vi "FT10_Log Tester Queue Data.vi"(10 "Queue in":refnum<queue>, 11 "Cluster in":T1) -> (3 "Cluster out":T1)   [LabVIEW 2015]
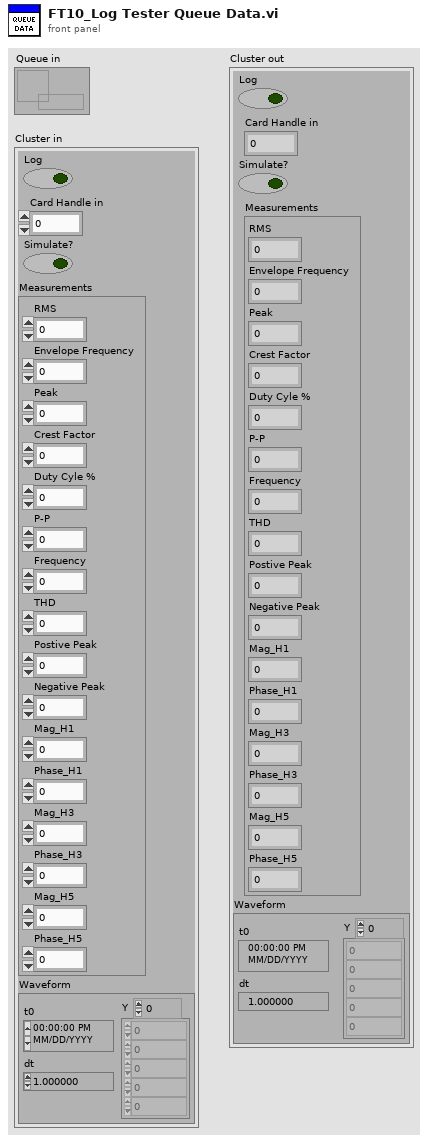
[diagram p1: front panel]
types:
  T1 = cluster{"Log":bool, "Card Handle in":u32, "Simulate?":bool, "Measurements":cluster{"RMS":dbl, "Envelope Frequency":dbl, "Peak":dbl, "Crest Factor":dbl, "Duty Cyle %":dbl, "P-P":dbl, "Frequency":dbl, "THD":dbl, "Postive Peak":dbl, "Negative Peak":dbl, "Mag_H1":dbl, "Phase_H1":dbl, "Mag_H3":dbl, "Phase_H3":dbl, "Mag_H5":dbl, "Phase_H5":dbl}, "Waveform":waveform(dbl)}
  T2 = cluster{"Time":timestamp, "Waveform":waveform(dbl), "Measurements":cluster{"RMS":dbl, "Envelope Frequency":dbl, "Peak":dbl, "Crest Factor":dbl, "Duty Cyle %":dbl, "P-P":dbl, "Frequency":dbl, "THD":dbl, "Postive Peak":dbl, "Negative Peak":dbl, "Mag_H1":dbl, "Phase_H1":dbl, "Mag_H3":dbl, "Phase_H3":dbl, "Mag_H5":dbl, "Phase_H5":dbl}}
  T3 = cluster{"RMS":dbl, "Envelope Frequency":dbl, "Peak":dbl, "Crest Factor":dbl, "Duty Cyle %":dbl, "P-P":dbl, "Frequency":dbl, "THD":dbl, "Postive Peak":dbl, "Negative Peak":dbl, "Mag_H1":dbl, "Phase_H1":dbl, "Mag_H3":dbl, "Phase_H3":dbl, "Mag_H5":dbl, "Phase_H5":dbl}
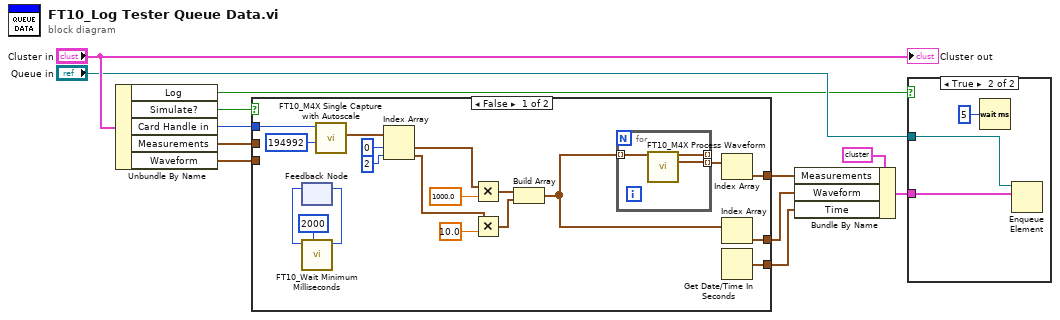
[diagram p0: block diagram]
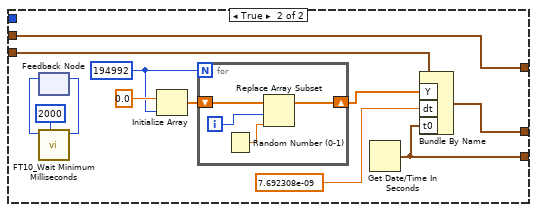
[diagram p3: hidden frame]
diagram:
  n1 = Unbundle By Name("Cluster in") -> ("Log"=w3:bool, "Simulate?"=w1:bool, "Card Handle in"=w2:u32, "Measurements"=w11:T3, "Waveform"=w12:waveform(dbl))
  n2 = case shown="False" w1 {
    tunnel: [w19 w46] -> w7
    tunnel: [w18 w41] -> w5
    tunnel: w2 -> [w17 _]
    tunnel: [w16 w35] -> w6
    tunnel: w11 -> [_ w46]
    tunnel: w12 -> [_ w42]
    frame False {
      n3 = feedback #1() -> (w13:u32)  [unwired: 1 in]
      n4 = call "FT10_Wait Minimum Milliseconds.vi"("Minimum ms wait"=u32 2000, "previous millisecond timer value in"=w13) -> ("millisecond timer value out"=w14:u32)  [unwired: 8 in, 1 out]
      n5 = feedback-in #1(w14) -> ()
      n6 = call "FT10_M4X Single Capture with Autoscale.vi"("memsize"=194992, "Card Handle in"=w17) -> ("Data"=w28:waveform(sgl)[])  [unwired: 8 in, 1 out]
      n7 = Index Array(array=w28, index #1=0 ("index"), index #2=2 ("index")) -> (element #1=w22:waveform(sgl), element #2=w21:waveform(sgl))
      n8 = Multiply(x=w22, y=1000.0) -> (x*y=w25:waveform(dbl))
      n9 = Multiply(x=w21, y=10.0) -> (x*y=w24:waveform(dbl))
      n10 = Build Array(w25, w24) -> (w20:waveform(dbl)[])
      n11 = for {
        tunnel: w20 -> [w32] mode=indexing
        tunnel: [w34] -> w23 mode=indexing
        tunnel: [w33] -> _ mode=indexing
        n12 = call "FT10_M4X Process Waveform.vi"("RF Waveform In"=w32) -> ("RF Waveform Out"=w33:waveform(sgl), "Measurements"=w34:T3)  [unwired: 12 in, 1 out]
      }
      n13 = Index Array(array=w23) -> (element=w19:T3)  [unwired: 1 in]
      n14 = Index Array(array=w20) -> (element=w18:waveform(dbl))  [unwired: 1 in]
      n15 = Get Date/Time In Seconds() -> (seconds since 1Jan1904=w16:timestamp)
    }
    frame True {
      w39 = 194992 ("memsize")
      n16 = feedback #2() -> (w43:u32)  [unwired: 1 in]
      n17 = call "FT10_Wait Minimum Milliseconds.vi"("Minimum ms wait"=u32 2000, "previous millisecond timer value in"=w43) -> ("millisecond timer value out"=w44:u32)  [unwired: 8 in, 1 out]
      n18 = feedback-in #2(w44) -> ()
      n19 = Initialize Array(0.0 ("element"), w39) -> (w38:dbl[])
      n20 = for {
        N: w39 -> [_]
        shift-right: [w49] -> w37
        shift-left: w38 -> [w50]
        i -> [w48]
        n21 = Random Number (0-1)() -> (number: 0 to 1=w47:dbl)
        n22 = Replace Array Subset(array=w50, new element=w47, index=w48) -> (w49:dbl[])
      }
      n23 = Get Date/Time In Seconds() -> (seconds since 1Jan1904=w35:timestamp)
      n24 = Bundle By Name(cluster=w42, "Y"=w37, "dt"=7.692308e-09, "t0"=w35) -> (w41:waveform(dbl))
    }
  }
  n25 = Bundle By Name(cluster=T2 {"Time"=timestamp(0 s since 1904-01-01), "Waveform"={"t0"=timestamp(0 s since 1904-01-01), "dt"=1.0, "Y"=[]}, "Measurements"={"RMS"=0.0, "Envelope Frequency"=0.0, "Peak"=0.0, "Crest Factor"=0.0, "Duty Cyle %"=0.0, "P-P"=0.0, "Frequency"=0.0, "THD"=0.0, "Postive Peak"=0.0, "Negative Peak"=0.0, "Mag_H1"=0.0, "Phase_H1"=0.0, "Mag_H3"=0.0, "Phase_H3"=0.0, "Mag_H5"=0.0, "Phase_H5"=0.0}}, "Measurements"=w7, "Waveform"=w5, "Time"=w6) -> (w8:T2)
  n26 = case shown="True" w3 {
    tunnel: w8 -> [_ w52]
    tunnel: "Queue in" -> [_ w53]
    frame False {
    }
    frame True {
      n27 = Wait (ms)(milliseconds to wait=u32 5) -> ()  [unwired: 1 out]
      n28 = Enqueue Element(queue=w53, element=w52) -> ()  [unwired: 2 in, 3 out]
    }
  }
  "Cluster out" <- "Cluster in"
